vi "Documentation Application Tool.vi"() -> ()   [LabVIEW 2016]
uses:
  <vilib>/ni/Tree/Tree Manager/Tree.lvclass
  States.ctl
  <vilib>/ni/Tree/Data Types/String/String.lvclass/String.ctl
  <vilib>/ni/Tree/Data Types/String/To String Tree Data.vi
  <vilib>/ni/Tree/Data Types/String/From String Tree Data.vi
  <vilib>/ni/Tree/Data Types/String/String.lvclass
  C:/Program Files/National Instruments/LabVIEW 2016/vi.lib/ni/Tree/Tree Data/Tree Data.lvclass
  <vilib>/ni/Tree/Tree Manager/API/Set Attribute.vi
  <vilib>/ni/Tree/Tree Manager/API/Set Meta Data.vi
  <vilib>/ni/Tree/Tree Manager/API/Get Name.vi
  <vilib>/ni/Tree/Tree Manager/API/Set Name.vi
  <vilib>/ni/Tree/Tree Manager/API/Set Attribute Tree Data.vi
  <vilib>/xml/Load XML File.vi
  <vilib>/ni/Tree/Tree Manager/API/List Roots.vi
  <vilib>/ni/Tree/Tree Manager/API/Get Attribute Tree Data.vi
  <vilib>/ni/Tree/Tree Manager/API/Get Meta Data.vi
  <vilib>/ni/Tree/Tree Manager/API/Delete Attribute Tree Data.vi
  <vilib>/ni/Tree/Tree Manager/API/Get Attribute.vi
  <vilib>/xml/NI_XML.lvlib
panel:
  in  "Load XML File":bool
  in  "XML File Path":path=path "C:/Git/rfic-reference-design-libraries-csharp/CodeReport.xml"
  in  "Load Search Directory":bool
  in  "Search Directory":path=path "C:/Git/rf-adv-reference-design-libraries-labview/Source/SG"
  in  "Code Modules":string(tree)
  in  "XML File":string(tree)
  out "Selected Element":string
  in  "Element Description":string
  in  "Copy":bool
  out "Selected XML Data":string
  in  "Cancel":bool
  in  "Apply All Unsaved":bool
  in  "Cancel All":bool
  in  "Apply":bool
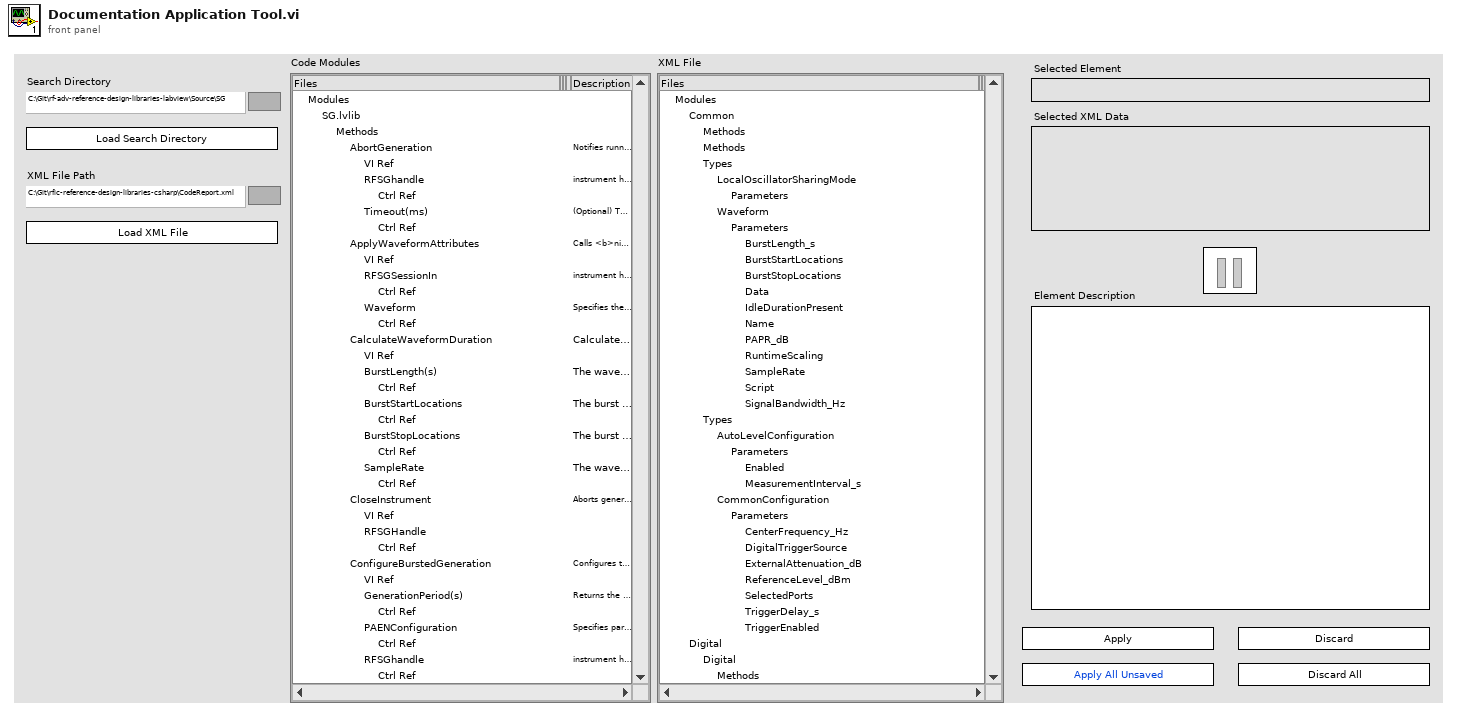
[diagram p1: front panel]
types:
  T1 = typedef "States.ctl" = enum16{"<Init>", "Wait for Event", "Update Code Modules Display", "Save Files", "<Shutdown>"}
  T2 = cluster{"LabVIEW Tree":refnum<data-value>, "XML Tree":refnum<data-value>, "References":refnum<vi>[], "Unsaved Items":variant, "Control Strings":string[], "Items to Save":string[]}
  T3 = enum32{"invalid VI type", "Standard VI", "Control VI", "Global VI", "Polymorphic VI", "Configuration VI", "SubSystem", "Facade VI", "Method VI", "Statechart Diagram VI"}
  T4 = enum16{"Left Button", "Center Button", "Right Button", "Window Close"}
  T5 = cluster{"Left Cell String":string, "Child Text":string[], "Child Tag":string, "Item Indent":i32, "Child Only?":bool, "Glyph Index":i32}[]
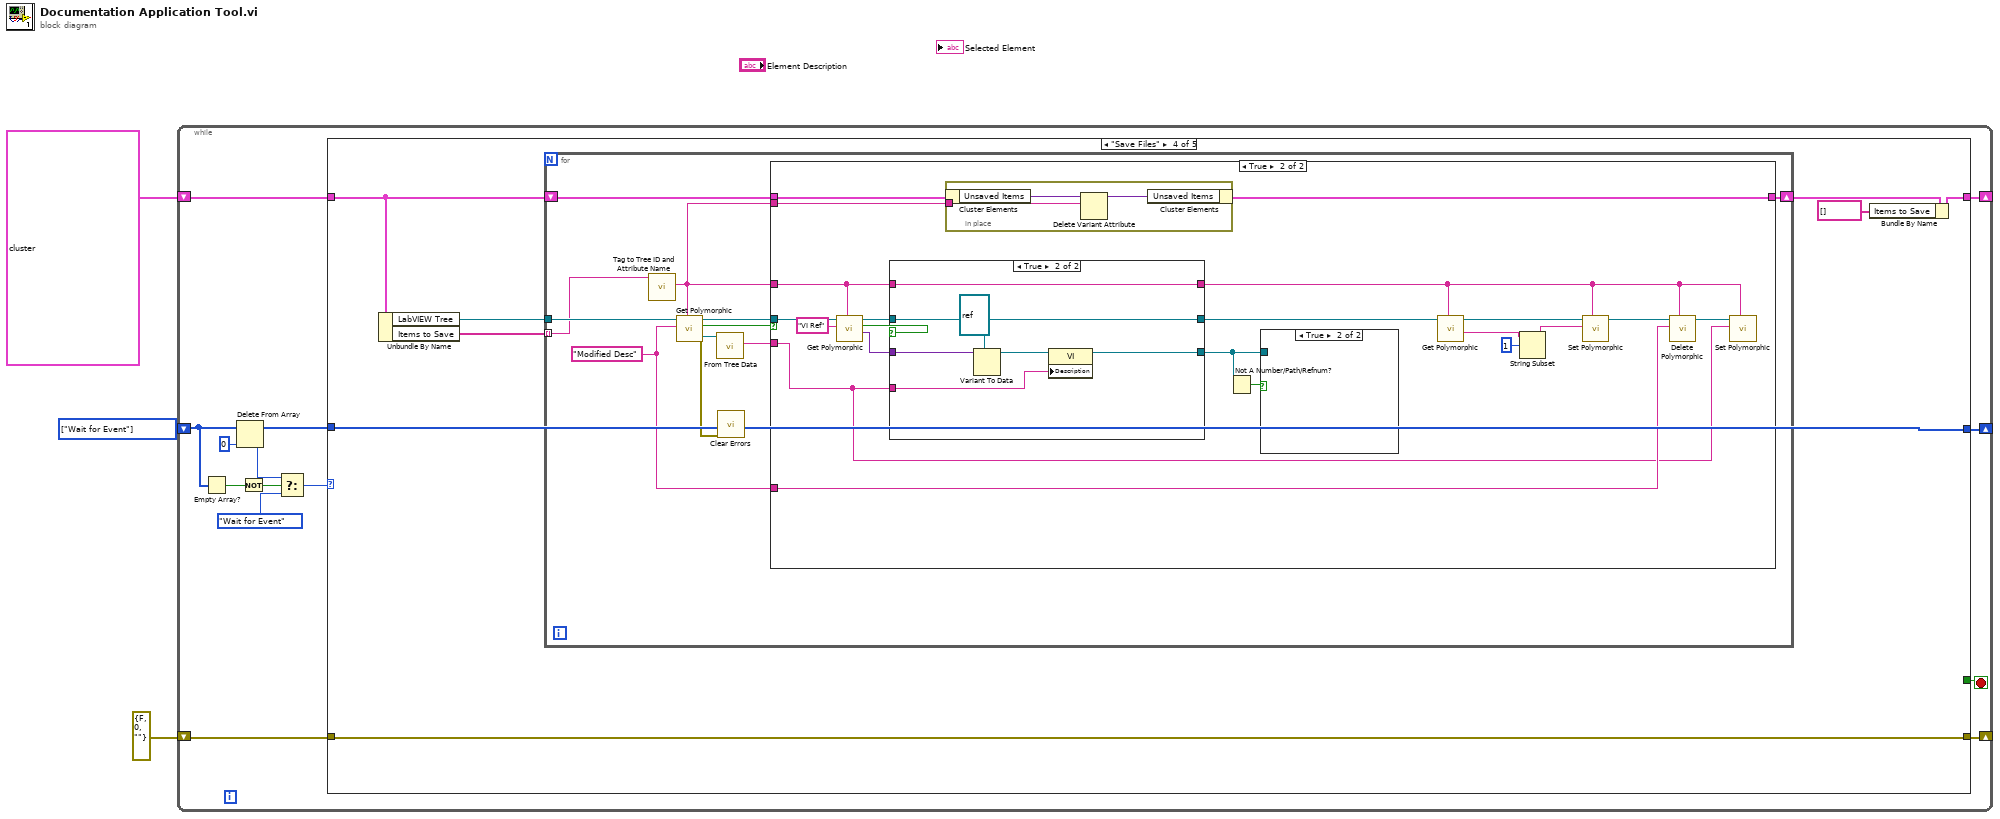
[diagram p0: block diagram]
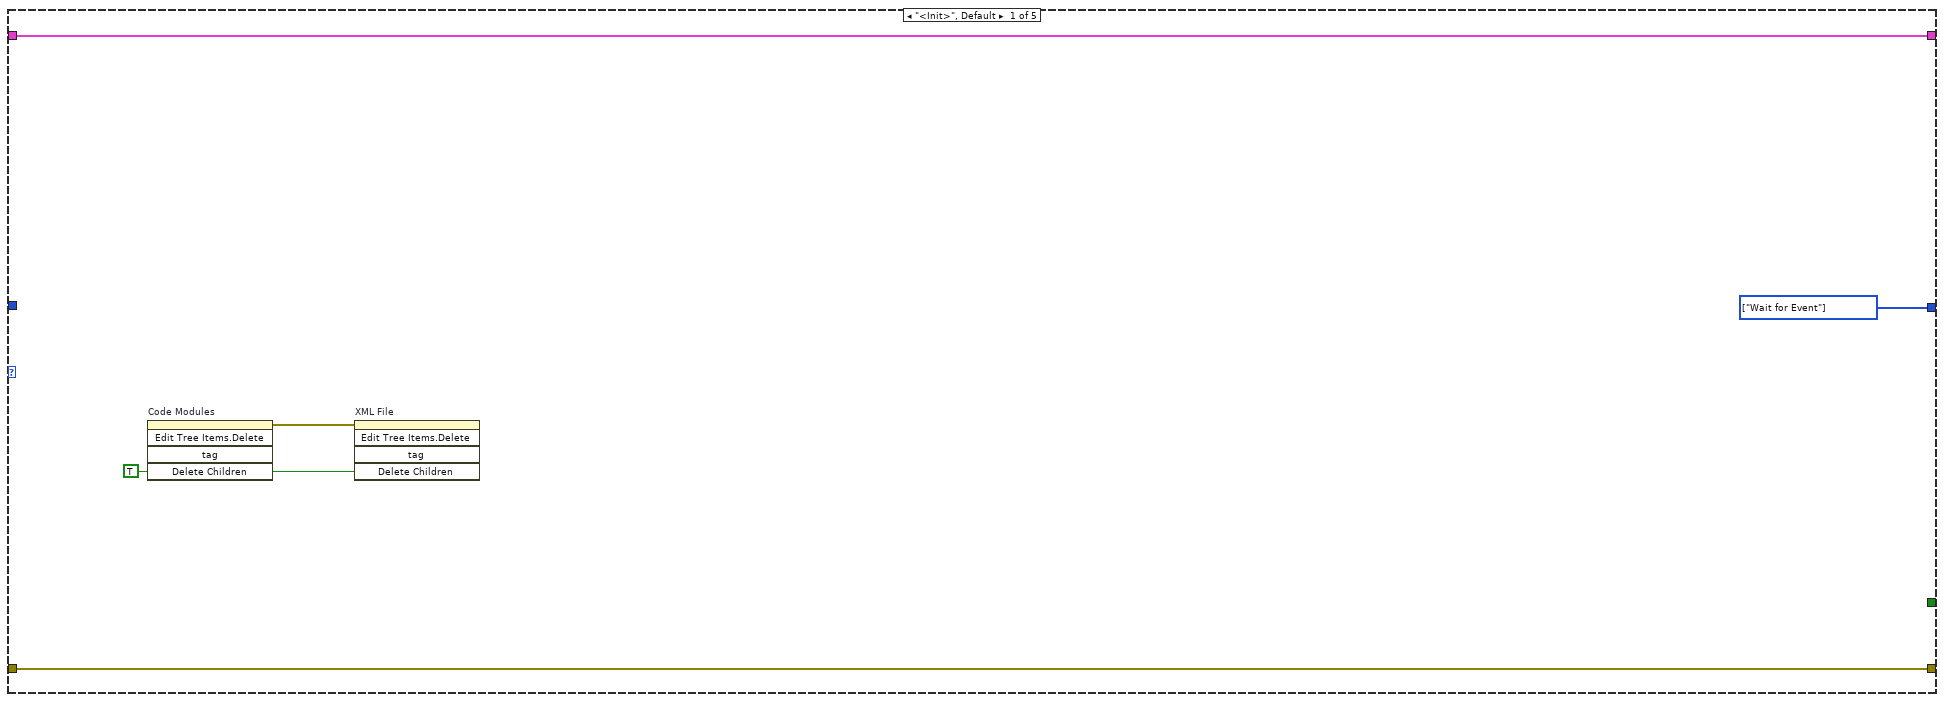
[diagram p2: hidden frame]
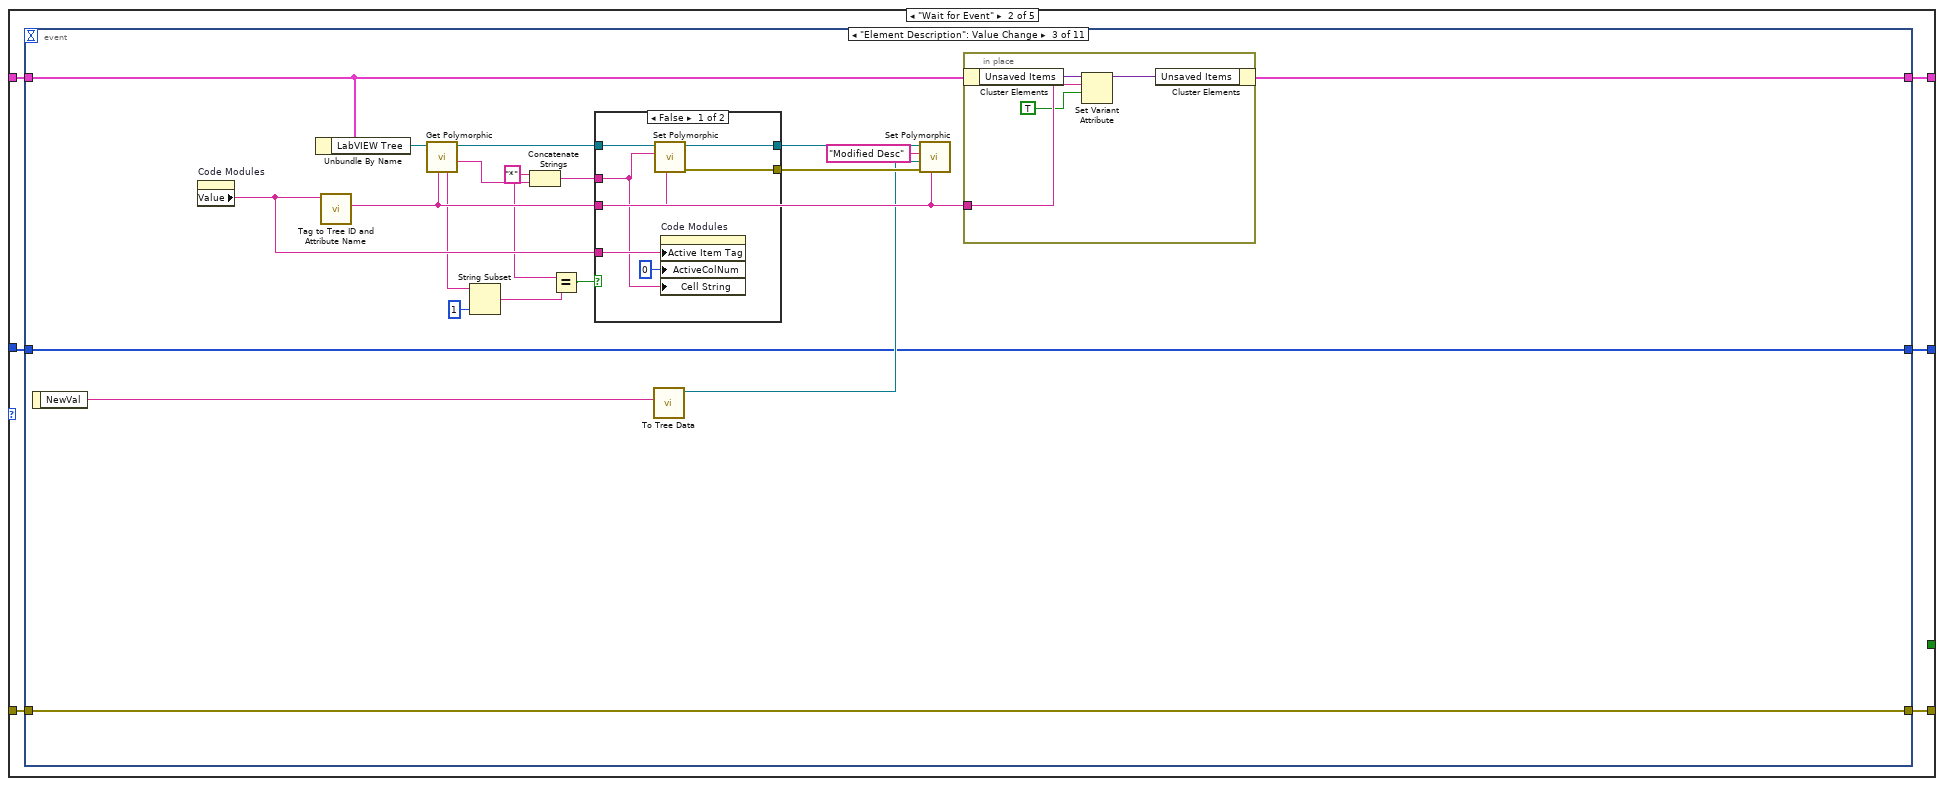
[diagram p3: hidden frame]
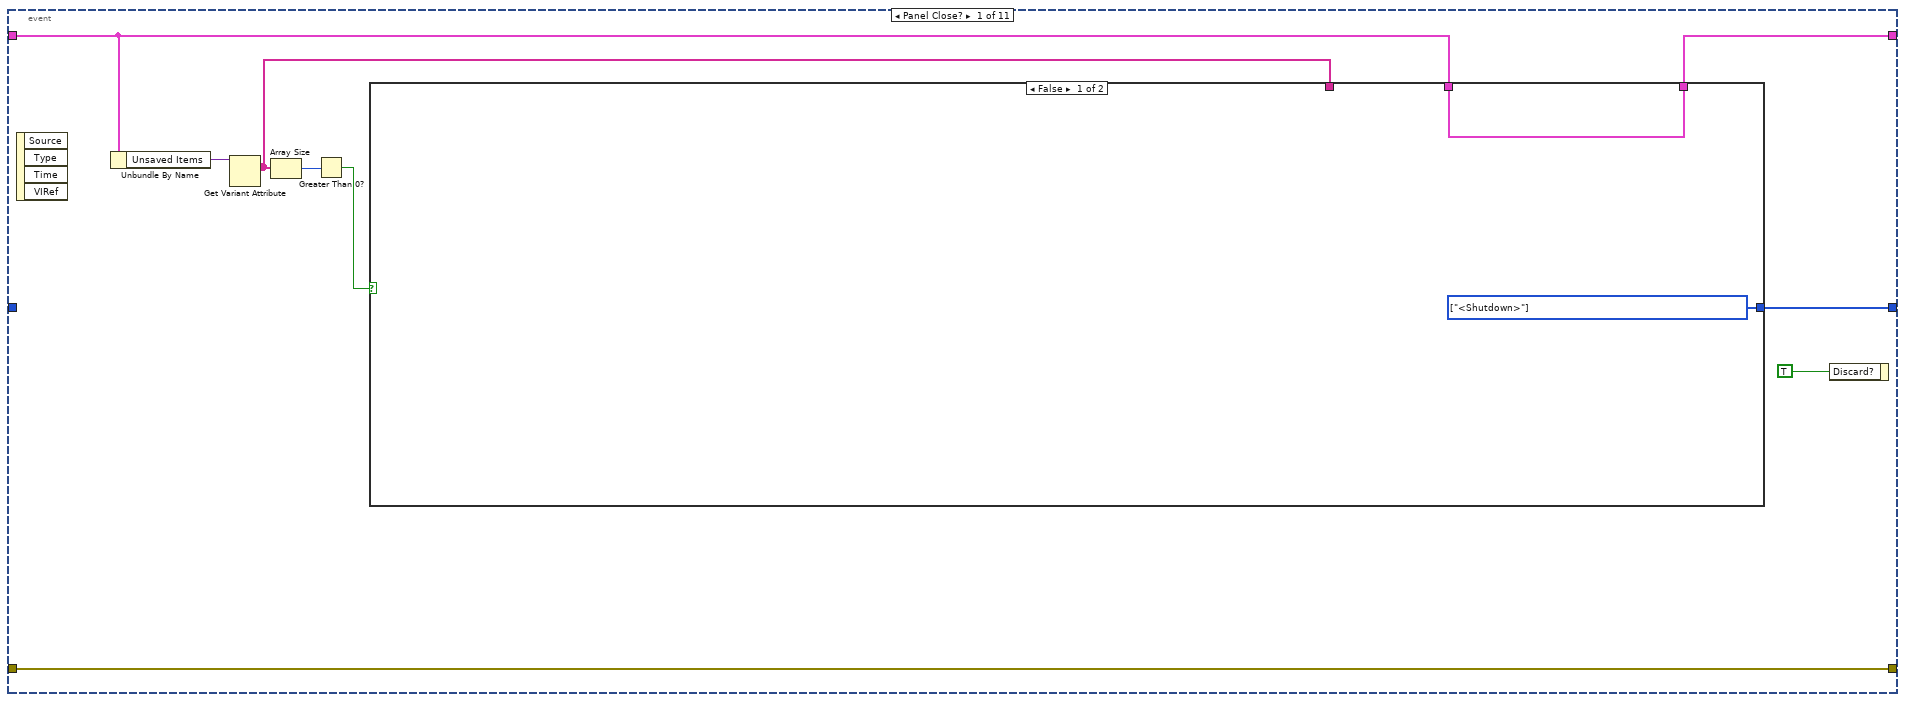
[diagram p4: hidden frame]
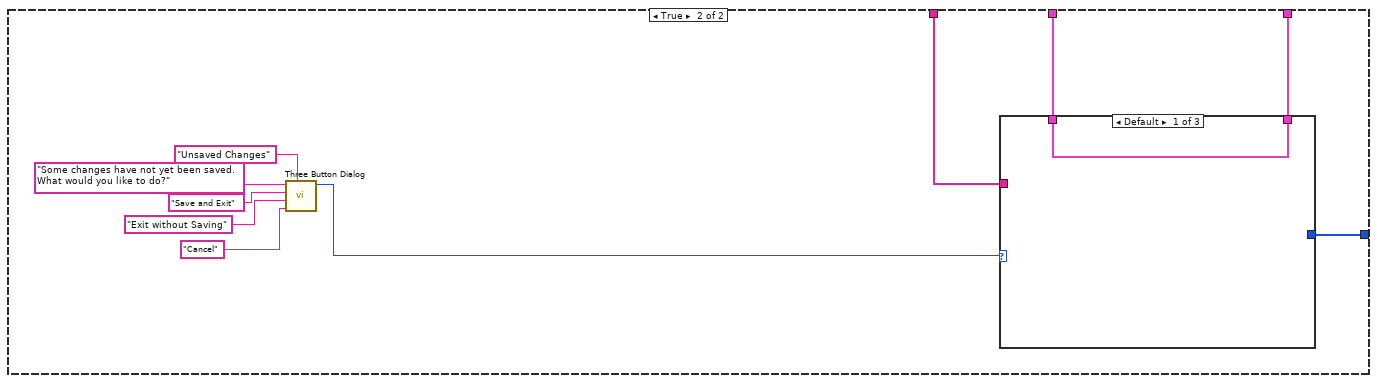
[diagram p5: hidden frame]
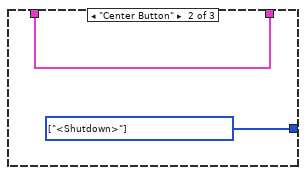
[diagram p6: hidden frame]
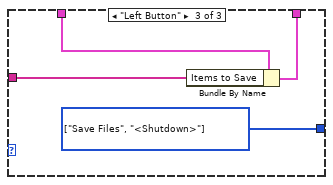
[diagram p7: hidden frame]
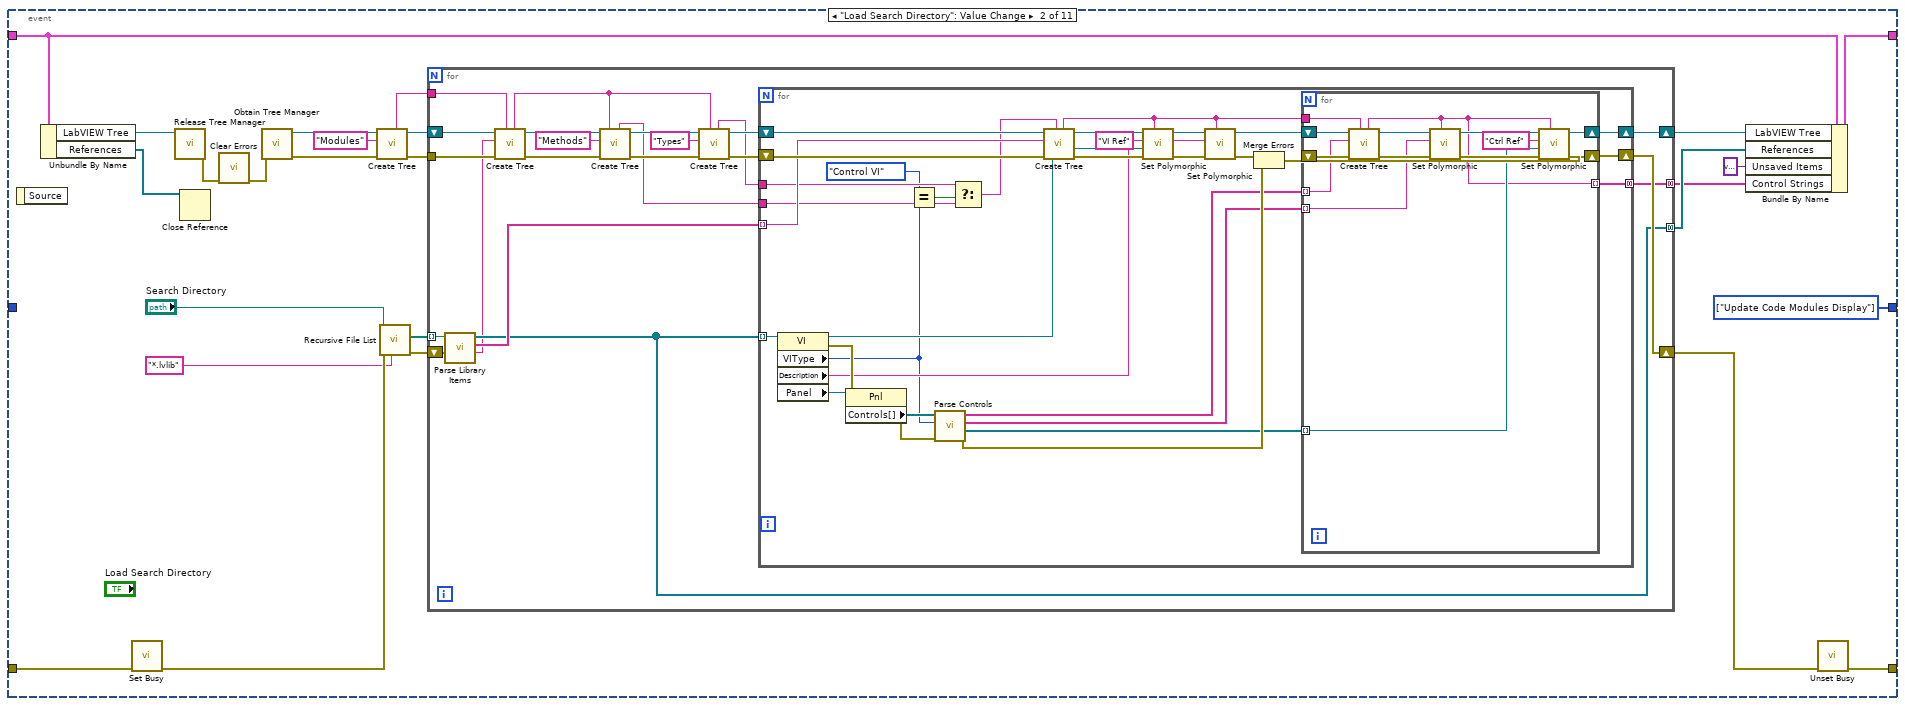
[diagram p8: hidden frame]
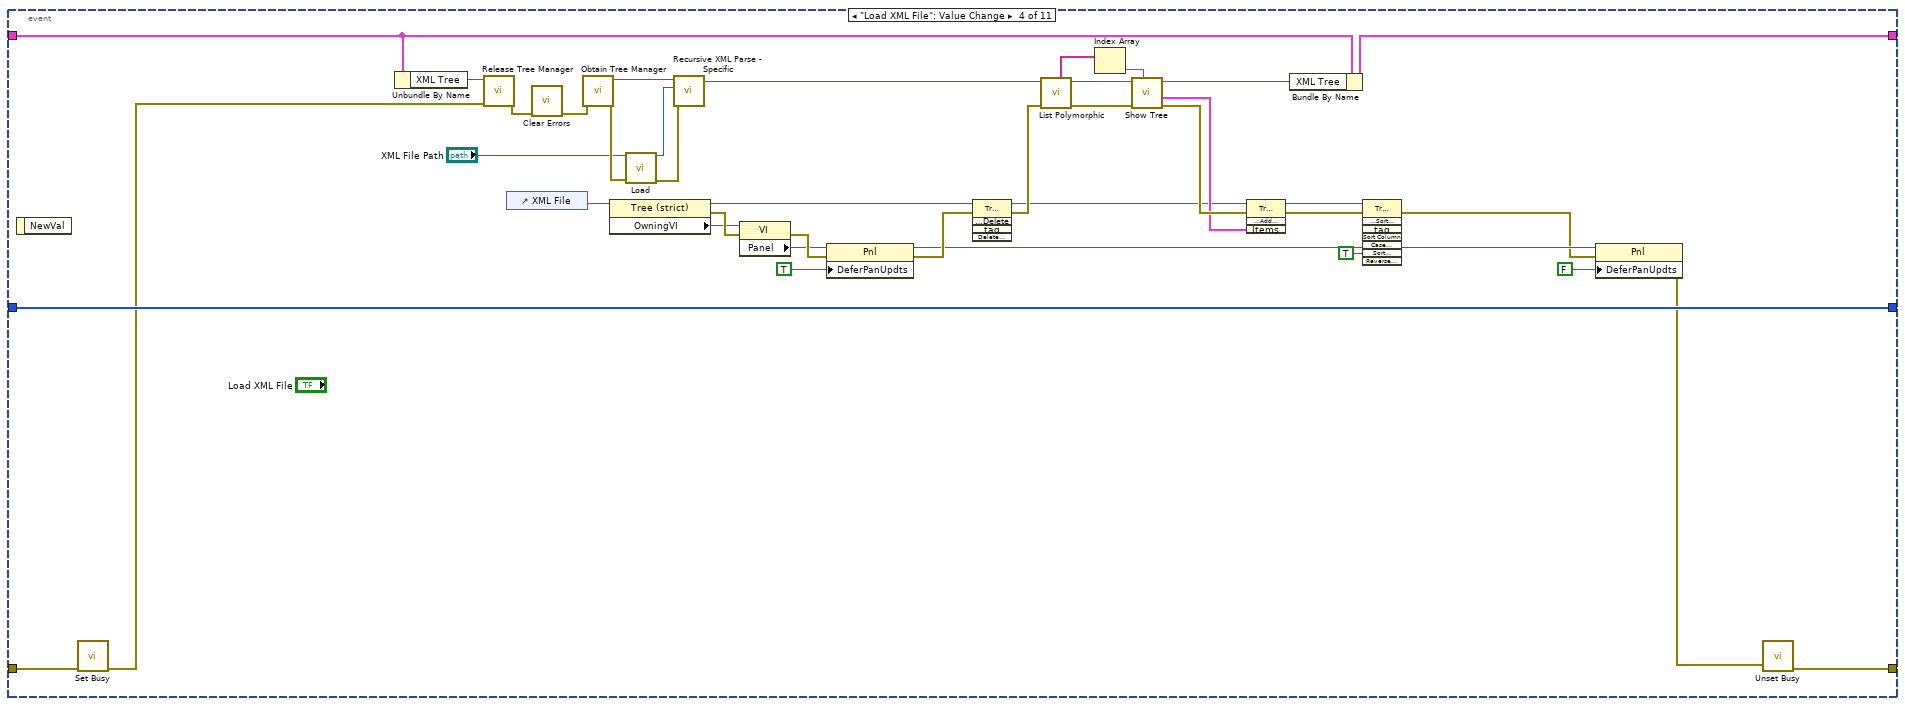
[diagram p10: hidden frame]
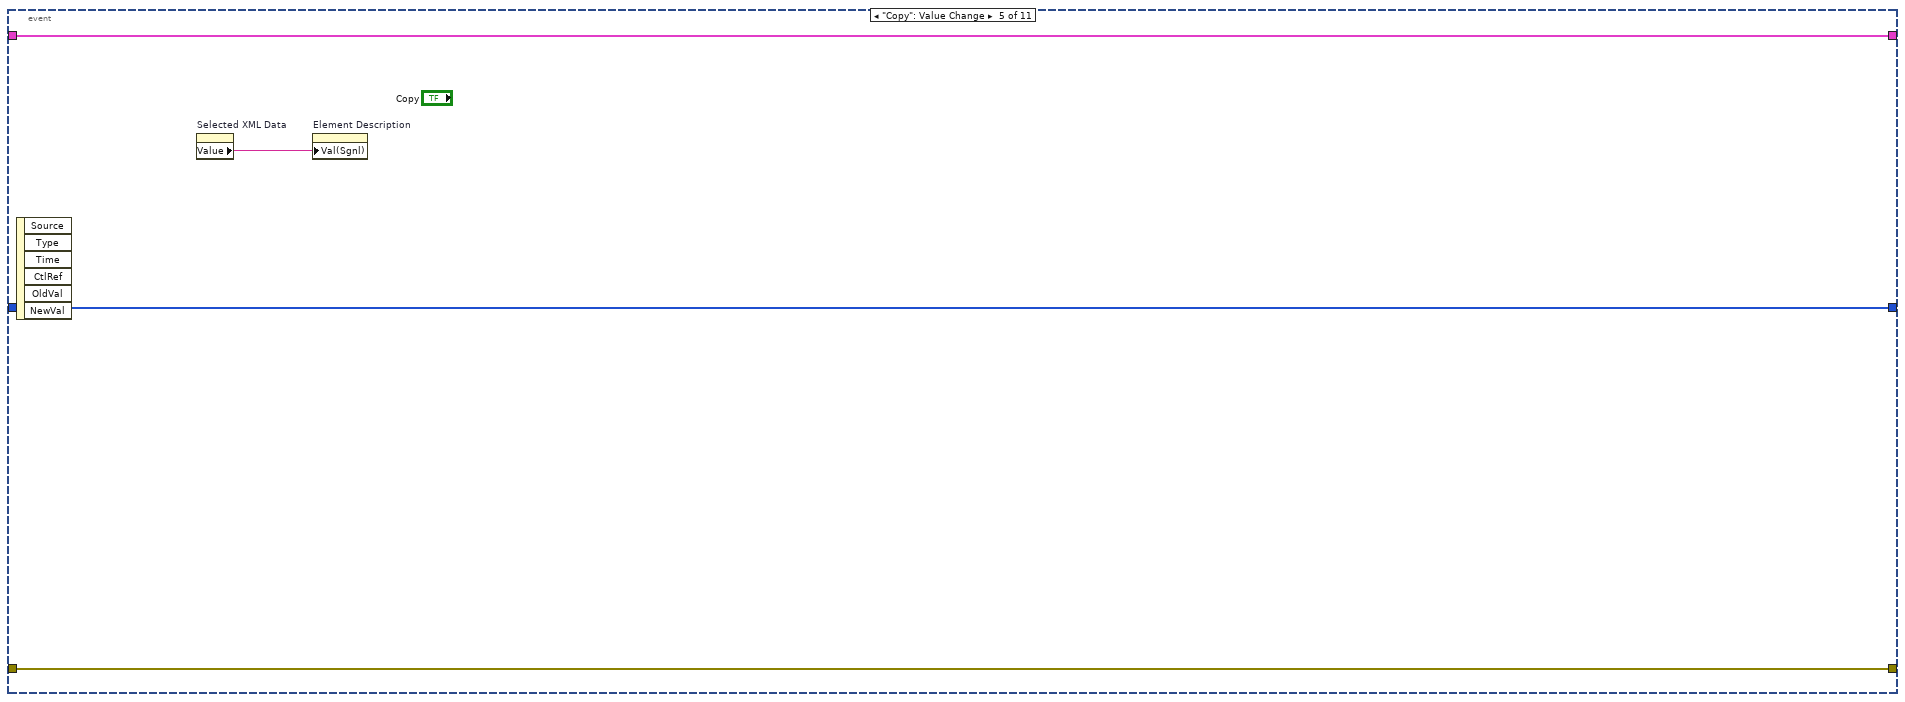
[diagram p11: hidden frame]
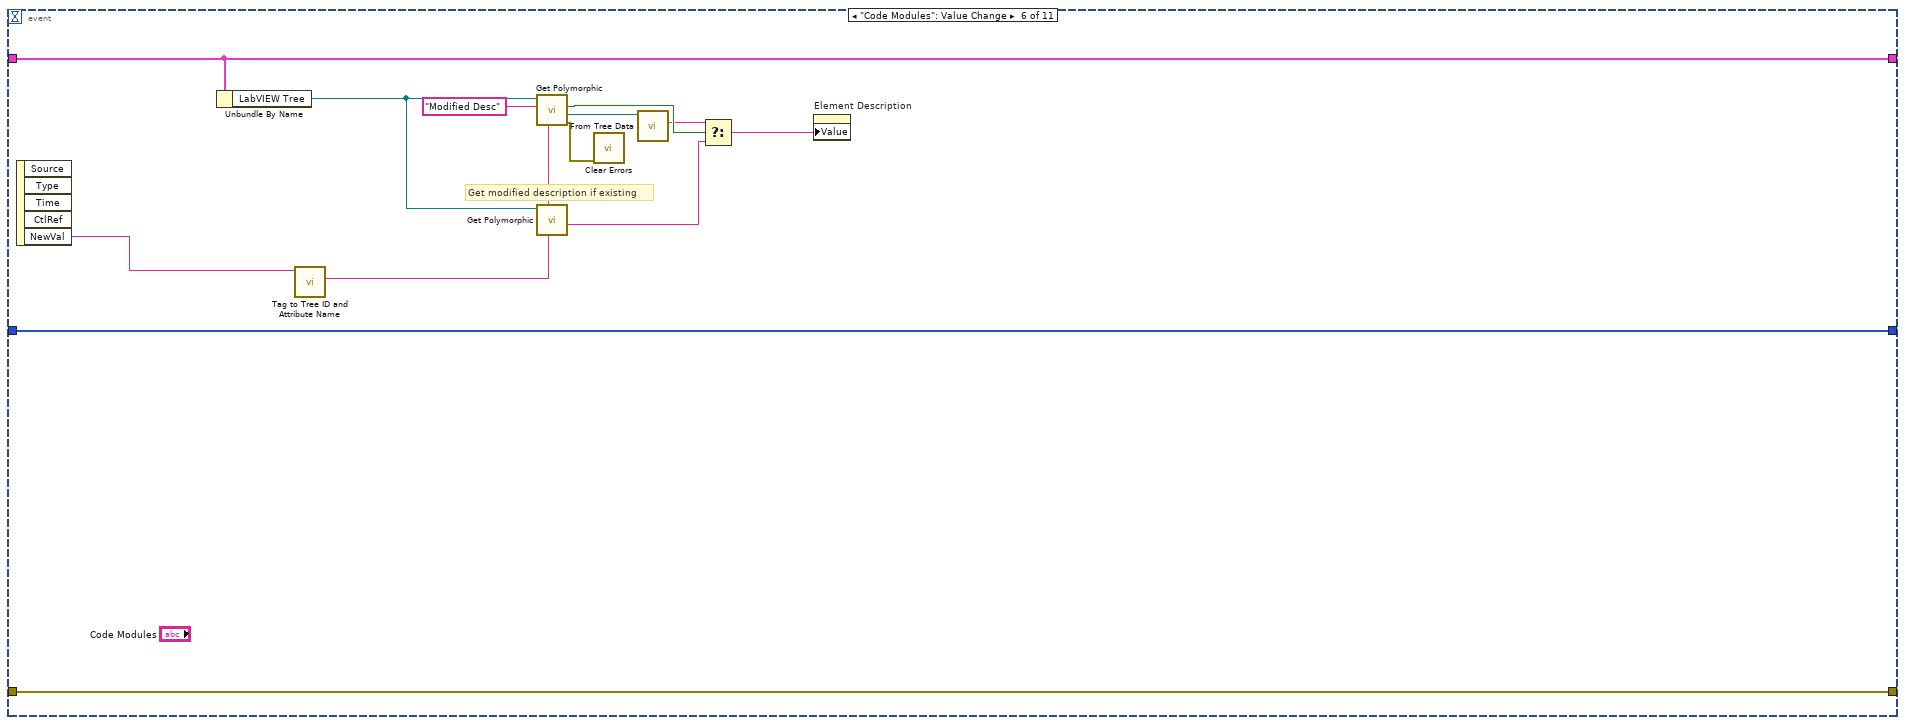
[diagram p12: hidden frame]
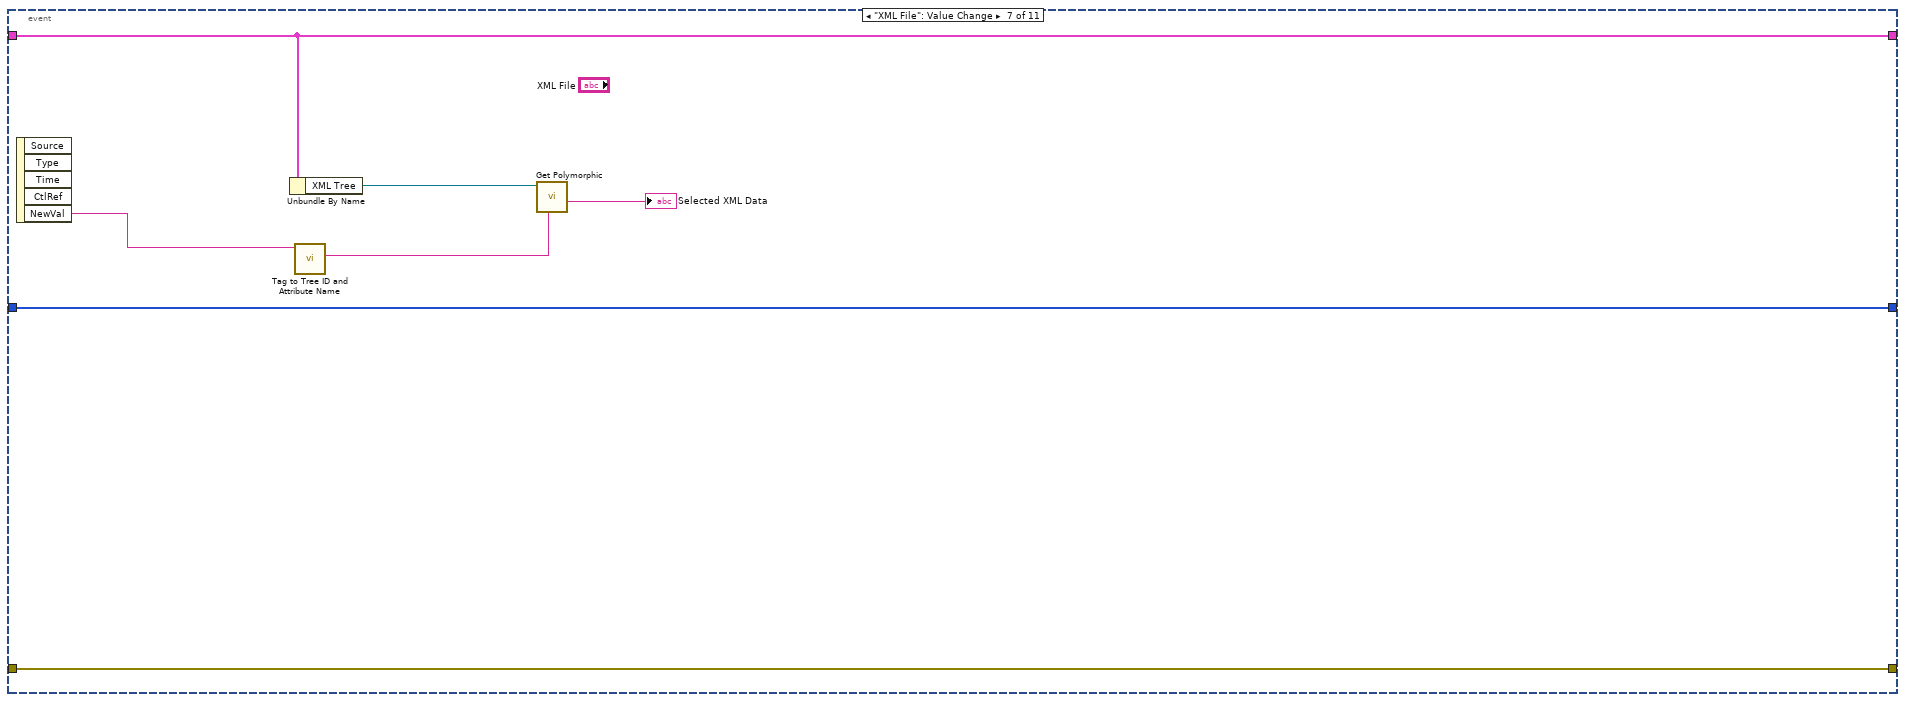
[diagram p13: hidden frame]
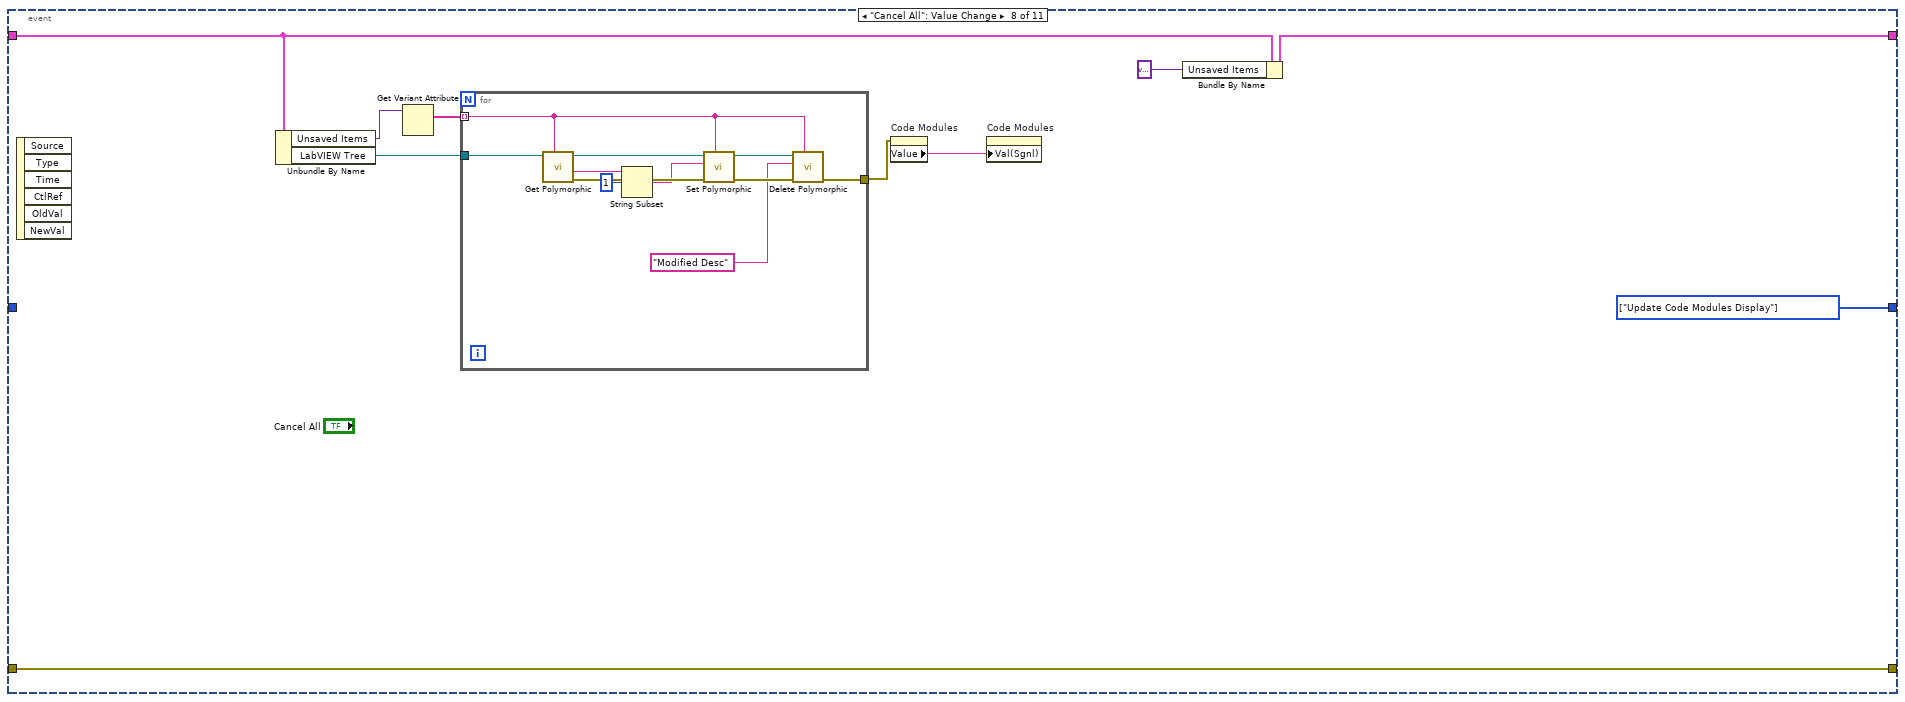
[diagram p14: hidden frame]
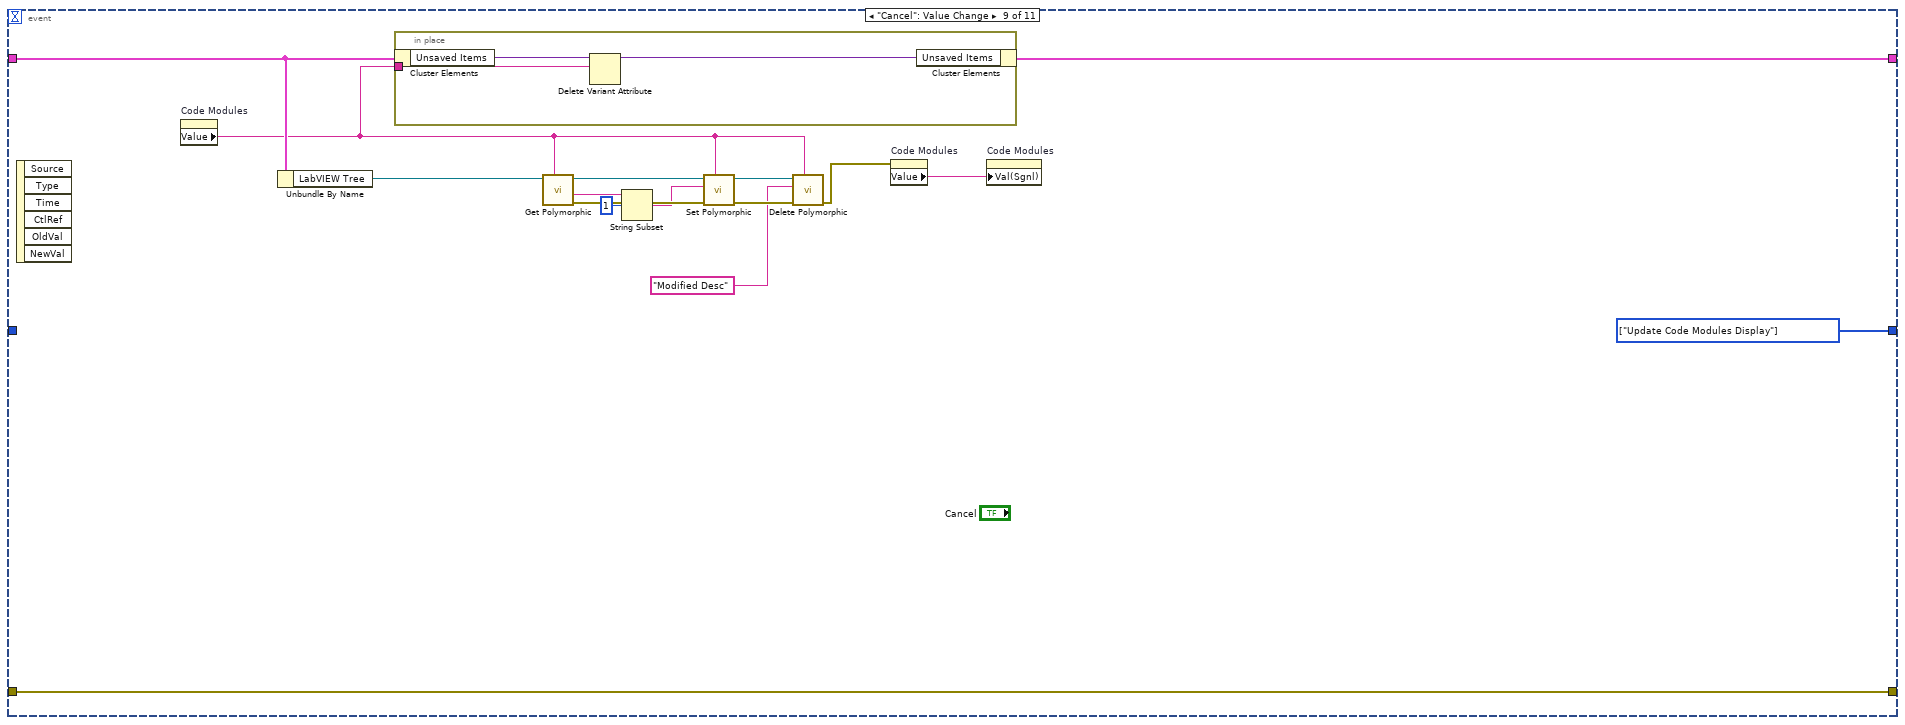
[diagram p15: hidden frame]
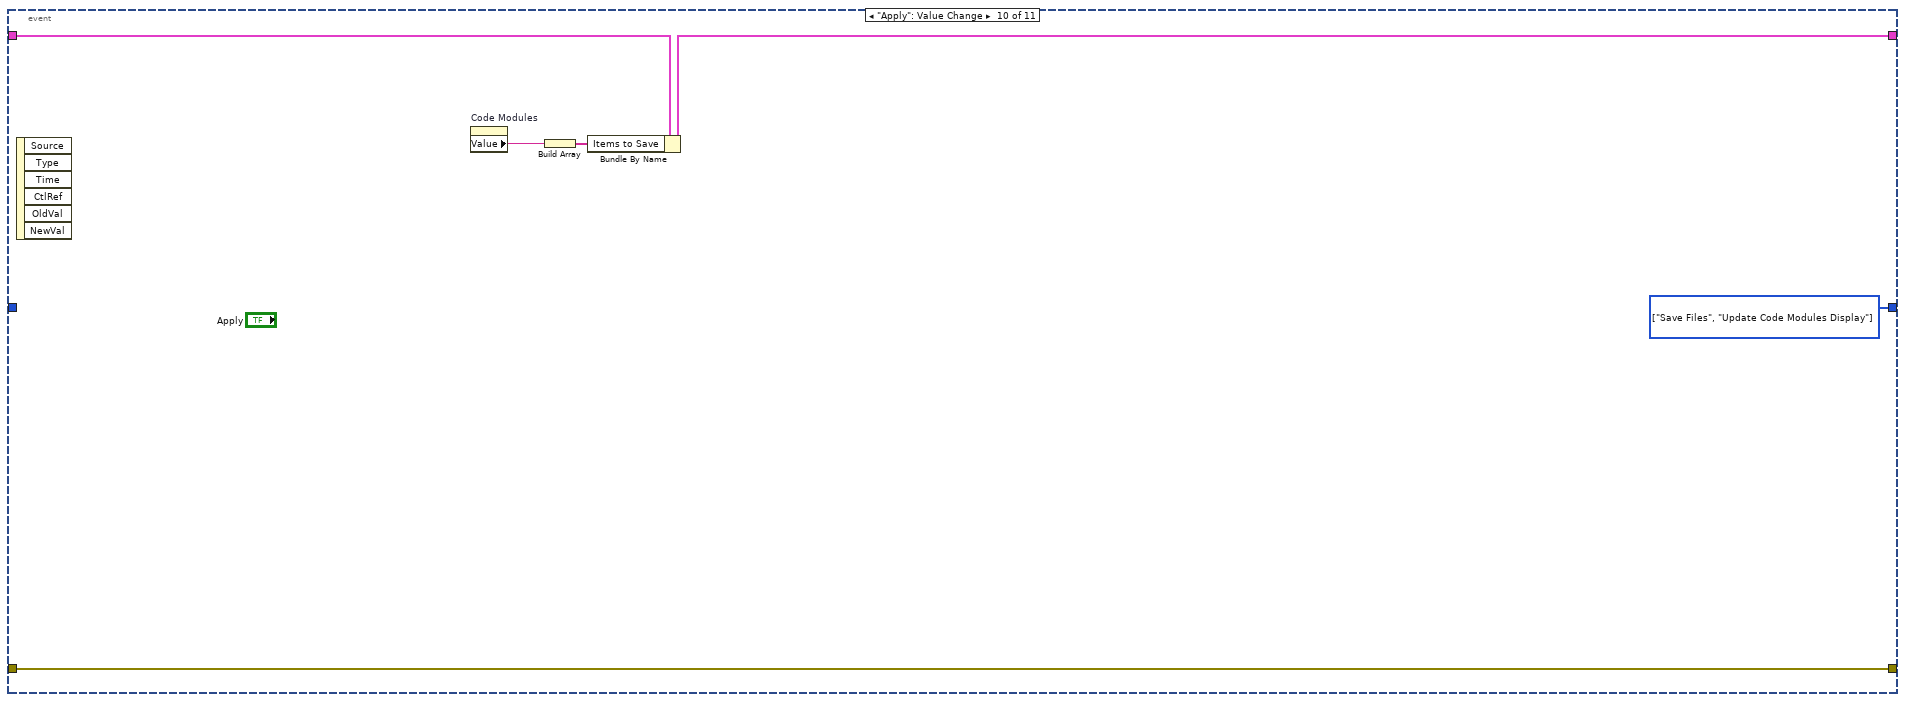
[diagram p16: hidden frame]
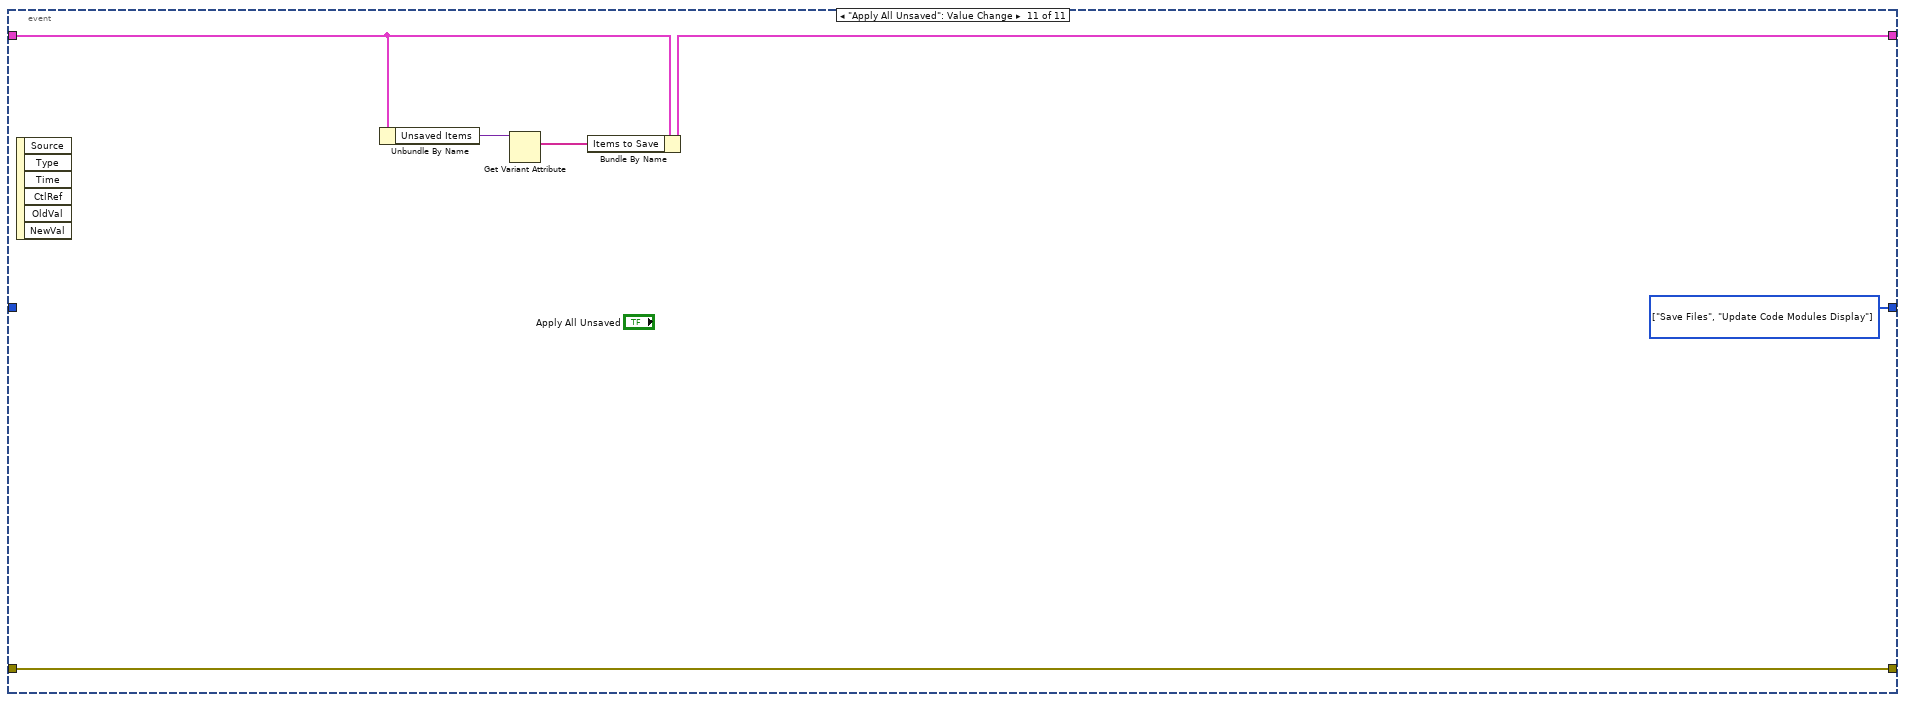
[diagram p17: hidden frame]
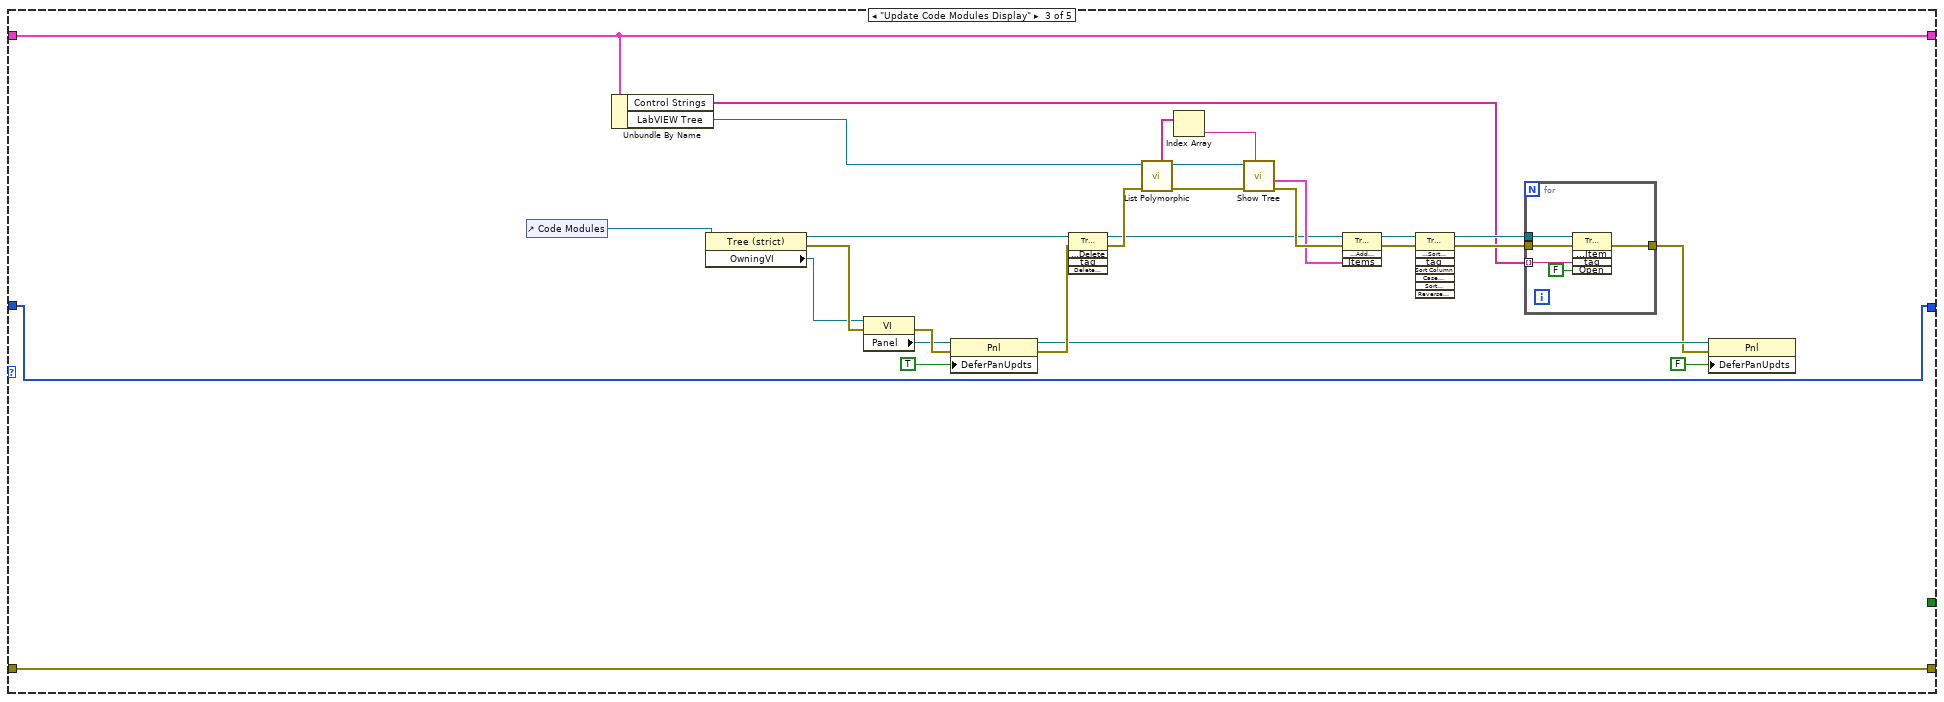
[diagram p18: hidden frame]
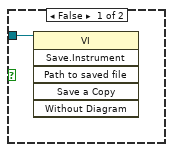
[diagram p20: hidden frame]
diagram:
  w1 = T1[] [enum."Wait for Event"] items=["<Init>", "Wait for Event", "Update Code Modules Display", "Save Files", "<Shutdown>"]
  n1 = while {
    shift-right: [w16] -> _
    shift-left: errorcluster {"status"=FALSE, "code"=0, "source"=""} ("error constant") -> [w17]
    shift-right: [w14] -> _
    shift-left: T2 {"LabVIEW Tree"=refnum, "XML Tree"=refnum, "References"=[], "Unsaved Items"=variant, "Control Strings"=[], "Items to Save"=[]} -> [w15]
    shift-right: [w5] -> _
    shift-left: w1 -> [w11]
    stop <- w4 stop-if-true
    n2 = Empty Array?(array=w11) -> (empty?=w10:bool)
    n3 = Delete From Array(array=w11, index=0) -> (deleted portion=w9:T1, array with subset deleted=w13:T1[])  [unwired: 1 in]
    n4 = Not(x=w10) -> (.not. x?=w8:bool)
    n5 = Select(t=w9, s=w8, f=States."Wait for Event") -> (s? t:f=w6:T1)
    n6 = case shown="\"Save Files\"" w6 {
      tunnel: w17 -> [w21 w28 w323 w336 w404]
      tunnel: [w21 w27 w323 w336 w404] -> w16
      tunnel: w15 -> [w18 w26 w315 w334 w401]
      tunnel: [w18 w25 w315 w331 w401] -> w14
      tunnel: w13 -> [_ w23 w296 w329 w402]
      tunnel: [w19 w24 w296 w329 w402] -> w5
      tunnel: [_ _ _ _ TRUE] -> w4
      frame "<Init>", Default {
        w19 = T1[] [enum."Wait for Event"] items=["<Init>", "Wait for Event", "Update Code Modules Display", "Save Files", "<Shutdown>"]
        w20 = TRUE ("Delete Children?")
        n7 = invoke on="Code Modules" class="Tree (strict)" method="Edit Tree Items.Delete"("Delete Children"=w20) -> (error out=w22:errorcluster)  [unwired: 4 in, 4 out]
        n8 = invoke on="XML File" class="Tree (strict)" method="Edit Tree Items.Delete"(error in=w22, "Delete Children"=w20) -> ()  [unwired: 3 in, 5 out]
      }
      frame "Wait for Event" {
        n9 = event shown="[2] \"Element Description\": Value Change" {
          selector: _ -> [_ _ _ _ _ _ _ _ _ _ _]
          dyn-events: _ -> [_ _ _ _ _ _ _ _ _ _ _]
          timeout: _ -> [_ _ _ _ _ _ _ _ _ _ _]
          tunnel: w28 -> [w37 w80 w168 w219 w223 w236 w243 w253 w280 w289 w295]
          tunnel: [w37 w79 w168 w186 w223 w236 w243 w253 w280 w289 w295] -> w27
          tunnel: w26 -> [w32 w63 w163 w205 w222 w235 w242 w252 w267 w287 w292]
          tunnel: [w31 w64 w162 w206 w222 w235 w242 w245 w265 w286 w293] -> w25
          tunnel: [w35 w60 w150 w188 w220 w224 w237 w250 w278 w288 w294] -> w24
          tunnel: w23 -> [_ _ w150 w188 w220 w224 w237 _ _ _ _]
          event Panel Close? {
            n10 = event-data() -> ()  [unwired: 1 in, 4 out]
            n11 = Unbundle By Name(w32) -> ("Unsaved Items"=w34:variant)
            n12 = Get Variant Attribute(Variant=w34) -> (names=w30:string[])  [unwired: 3 in, 3 out]
            n13 = Array Size(array=w30) -> (size(s)=w33:i32)
            n14 = Greater Than 0?(x=w33) -> (x > 0?=w29:bool)
            n15 = case shown="False" w29 {
              tunnel: [w38 w49] -> w35
              tunnel: w32 -> [w39 w47]
              tunnel: [w39 w46] -> w31
              tunnel: w30 -> [_ w45]
              frame False {
                w38 = T1[] [enum."<Shutdown>"] items=["<Init>", "Wait for Event", "Update Code Modules Display", "Save Files", "<Shutdown>"]
              }
              frame True {
                n16 = call <vilib>:"Three Button Dialog.vi"("Window Title (\"\")"="Unsaved Changes" ("Window Title (\"\")"), "Right Button Text (\"Cancel\")"="Cancel" ("Right Button Text (\"Cancel\")"), "Center Button Text (\"No\")"="Exit without Saving" ("Center Button Text (\"No\")"), "Left Button Text (\"Yes\")"="Save and Exit" ("Left Button Text (\"Yes\")"), "message"="Some changes have not yet been saved. What would you like to do?") -> ("Which Button?"=w48:T4)  [unwired: 6 in]
                n17 = case shown="Default" w48 {
                  tunnel: [_ w52 w56] -> w49
                  tunnel: w47 -> [w50 w51 w55]
                  tunnel: [w50 w51 w54] -> w46
                  tunnel: w45 -> [_ _ w53]
                  frame Default {
                  }
                  frame "Center Button" {
                    w52 = T1[] [enum."<Shutdown>"] items=["<Init>", "Wait for Event", "Update Code Modules Display", "Save Files", "<Shutdown>"]
                  }
                  frame "Left Button" {
                    w56 = T1[] [enum."Save Files", enum."<Shutdown>"] items=["<Init>", "Wait for Event", "Update Code Modules Display", "Save Files", "<Shutdown>"]
                    n18 = Bundle By Name(cluster=w55, "Items to Save"=w53) -> (w54:T2)
                  }
                }
              }
            }
            n19 = event-data("Discard?"=TRUE) -> ()  [unwired: 1 in, 1 out]
          }
          event "Load Search Directory": Value Change {
            w60 = T1[] [enum."Update Code Modules Display"] items=["<Init>", "Wait for Event", "Update Code Modules Display", "Save Files", "<Shutdown>"]
            n20 = event-data() -> ()  [unwired: 1 in, 1 out]
            n21 = Unbundle By Name(w63) -> ("LabVIEW Tree"=w69:refnum<data-value>, "References"=w59:refnum<vi>[])
            n22 = call <vilib>:"Set Busy.vi"("error in (no error)"=w80) -> ("error out"=w74:errorcluster)  [unwired: 9 in, 1 out]
            n23 = call <vilib>:"Release Tree Manager.vi"("Tree"=w69) -> ("Error Out"=w78:errorcluster)  [unwired: 10 in]
            n24 = Close Reference(reference=w59) -> ()  [unwired: 1 in, 1 out]
            n25 = call <vilib>:"Clear Errors.vi"("error in (no error)"=w78) -> ("error out"=w77:errorcluster)  [unwired: 5 in, 1 out]
            n26 = call <vilib>:"Obtain Tree Manager.vi"("Error In"=w77) -> ("Error Out"=w76:errorcluster, "Tree"=w68:refnum<data-value>)  [unwired: 9 in]
            n27 = call <vilib>:"Create Tree.vi"("Error In"=w76, "Name"="Modules", "Tree Manager"=w68) -> ("Error Out"=w75:errorcluster, "Tree Manager"=w65:refnum<data-value>, "Unique ID"=w66:string)  [unwired: 6 in]
            n28 = call <vilib>:"Recursive File List.vi"("pattern"="*.lvlib", "error in (no error)"=w74, "Folder Path"="Search Directory") -> ("error out"=w81:errorcluster, "All Files in Dir"=w70:path[])  [unwired: 4 in, 3 out]
            n29 = for {
              tunnel: w70 -> [w97] mode=indexing
              shift-right: [w98] -> w73
              shift-left: w81 -> [w103]
              tunnel: w66 -> [w92]
              tunnel: w75 -> [w102]
              tunnel: [w95] -> w62 mode=concatenating
              shift-right: [w83] -> w61
              shift-left: w65 -> [w94]
              tunnel: [w82] -> w57 mode=concatenating
              n30 = call "Parse Library Items.vi"("error in (no error)"=w103, "Library Path"=w97) -> ("Display Name"=w93:string, "File Names"=w96:string[], "References"=w95:refnum<vi>[])  [unwired: 6 in, 1 out]
              n31 = call <vilib>:"Create Tree.vi"("Parent ID (empty)"=w92, "Error In"=w102, "Name"=w93, "Tree Manager"=w94) -> ("Error Out"=w101:errorcluster, "Tree Manager"=w90:refnum<data-value>, "Unique ID"=w91:string)  [unwired: 5 in]
              n32 = call <vilib>:"Create Tree.vi"("Parent ID (empty)"=w91, "Error In"=w101, "Name"="Methods", "Tree Manager"=w90) -> ("Error Out"=w100:errorcluster, "Tree Manager"=w89:refnum<data-value>, "Unique ID"=w85:string)  [unwired: 5 in]
              n33 = call <vilib>:"Create Tree.vi"("Parent ID (empty)"=w91, "Error In"=w100, "Name"="Types", "Tree Manager"=w89) -> ("Error Out"=w99:errorcluster, "Tree Manager"=w86:refnum<data-value>, "Unique ID"=w84:string)  [unwired: 5 in]
              n34 = for {
                tunnel: w95 -> [w126] mode=indexing
                tunnel: w96 -> [w120] mode=indexing
                tunnel: w85 -> [w117]
                tunnel: w84 -> [w118]
                shift-right: [w107] -> w83
                shift-left: w86 -> [w121]
                shift-right: [w127] -> w98
                shift-left: w99 -> [w134]
                tunnel: [w104] -> w82 mode=concatenating
                n35 = property class="VI"(reference=w126) -> (reference out=w112:refnum<vi>, error out=w135:errorcluster, "VIType"=w105:T3, "Description"=w114:string, "Panel"=w106:refnum<vi>)  [unwired: 1 in]
                n36 = property class="Pnl"(reference=w106, error in=w135) -> (error out=w130:errorcluster, "Controls[]"=w125:refnum<vi>[])  [unwired: 1 out]
                n37 = Equal?(x=T3."Control VI" ("y"), y=w105) -> (x = y?=w119:bool)
                n38 = call "Parse Controls.vi"("error in (no error)"=w130, "VI Type"=w105, "Controls[]"=w125) -> ("error out"=w128:errorcluster, "References"=w122:refnum<vi>[], "Control Descriptions"=w123:string[], "Control Names"=w124:string[])  [unwired: 5 in]
                n39 = Select(t=w118, s=w119, f=w117) -> (s? t:f=w115:string)
                n40 = call <vilib>:"Create Tree.vi"("Parent ID (empty)"=w115, "Error In"=w134, "Name"=w120, "Tree Manager"=w121) -> ("Error Out"=w133:errorcluster, "Tree Manager"=w111:refnum<data-value>, "Unique ID"=w108:string)  [unwired: 5 in]
                n41 = call-poly <vilib>:"Set Polymorphic.vi"("Tree ID"=w108, "Error In"=w133, "Attribute Value"=w112, "Attribute Name"="VI Ref", "Tree Manager"=w111) -> ("Error Out"=w132:errorcluster, "Tree Manager"=w110:refnum<data-value>)  [unwired: 4 in, 1 out]
                n42 = call-poly <vilib>:"Set Polymorphic.vi"("Tree ID"=w108, "Error In"=w132, "Meta Data"=w114, "Tree Manager"=w110) -> ("Error Out"=w131:errorcluster, "Tree Manager"=w109:refnum<data-value>)  [unwired: 6 in]
                n43 = Merge Errors(w131, w128) -> (w129:errorcluster)
                n44 = for {
                  tunnel: w124 -> [w143] mode=indexing
                  tunnel: w123 -> [w142] mode=indexing
                  tunnel: w122 -> [w137] mode=indexing
                  shift-right: [w146] -> w127
                  shift-left: w129 -> [w149]
                  tunnel: w108 -> [w144]
                  shift-right: [w139] -> w107
                  shift-left: w109 -> [w145]
                  tunnel: [w136] -> w104 mode=indexing
                  n45 = call <vilib>:"Create Tree.vi"("Parent ID (empty)"=w144, "Error In"=w149, "Name"=w143, "Tree Manager"=w145) -> ("Error Out"=w148:errorcluster, "Tree Manager"=w141:refnum<data-value>, "Unique ID"=w136:string)  [unwired: 5 in]
                  n46 = call-poly <vilib>:"Set Polymorphic.vi"("Tree ID"=w136, "Error In"=w148, "Meta Data"=w142, "Tree Manager"=w141) -> ("Error Out"=w147:errorcluster, "Tree Manager"=w140:refnum<data-value>)  [unwired: 6 in]
                  n47 = call-poly <vilib>:"Set Polymorphic.vi"("Tree ID"=w136, "Error In"=w147, "Attribute Value"=w137, "Attribute Name"="Ctrl Ref", "Tree Manager"=w140) -> ("Error Out"=w146:errorcluster, "Tree Manager"=w139:refnum<data-value>)  [unwired: 4 in, 1 out]
                }
              }
            }
            n48 = Bundle By Name(cluster=w63, "LabVIEW Tree"=w61, "References"=w62, "Unsaved Items"=variant, "Control Strings"=w57) -> (w64:T2)
            n49 = call <vilib>:"Unset Busy.vi"("error in (no error)"=w73) -> ("error out"=w79:errorcluster)  [unwired: 10 in]
          }
          event "Element Description": Value Change {
            w152 = "*" ("string")
            n50 = event-data() -> ("NewVal"=w158:string)  [unwired: 1 in]
            n51 = property on="Code Modules" class="Tree (strict)"() -> ("Value"=w164:string)  [unwired: 2 in, 2 out]
            n52 = Unbundle By Name(w163) -> ("LabVIEW Tree"=w166:refnum<data-value>)
            n53 = call <vilib>:"Tag to Tree ID and Attribute Name.vi"("Tag"=w164) -> ("Tree ID"=w160:string)  [unwired: 8 in, 2 out]
            n54 = call-poly <vilib>:"Get Polymorphic.vi"("Tree ID"=w160, "Tree Manager"=w166) -> ("Name"=w156:string, "Tree Manager"=w165:refnum<data-value>)  [unwired: 7 in, 1 out]
            n55 = String Subset(string=w156, length (rest)=1 ("length (rest)")) -> (substring=w153:string)  [unwired: 1 in]
            n56 = Concatenate Strings(w152, w156) -> (w154:string)
            n57 = Equal?(x=w152, y=w153) -> (x = y?=w151:bool)
            n58 = case shown="False" w151 {
              tunnel: [w175 _] -> w167
              tunnel: w165 -> [w174 w176]
              tunnel: w164 -> [w173 _]
              tunnel: [w171 w176] -> w161
              tunnel: w160 -> [w170 _]
              tunnel: w154 -> [w169 _]
              frame False {
                n59 = call-poly <vilib>:"Set Polymorphic.vi"("Tree ID"=w170, "Name"=w169, "Tree Manager"=w174) -> ("Error Out"=w175:errorcluster, "Tree Manager"=w171:refnum<data-value>)  [unwired: 7 in]
                n60 = property on="Code Modules" class="Tree (strict)"("Active Item Tag"=w173, "ActiveColNum"=0 ("Active Cell:Active Column Number"), "Cell String"=w169) -> ()  [unwired: 2 in, 2 out]
              }
              frame True {
              }
            }
            n61 = call-poly <vilib>:"To Tree Data.vi"("String"=w158) -> ("String Tree Data"=w157:refnum<class "String.lvclass">)  [unwired: 10 in]
            n62 = call-poly <vilib>:"Set Polymorphic.vi"("Tree ID"=w160, "Error In"=w167, "Attribute Value"=w157, "Attribute Name"="Modified Desc", "Tree Manager"=w161) -> ()  [unwired: 4 in, 3 out]
            n63 = in-place {
              in-place-border: w160 -> [w179]
              n64 = in-place-cluster #1(w163) -> ("Unsaved Items"=w180:variant)
              n65 = Set Variant Attribute(Variant=w180, name=w179, value=TRUE) -> (Variant out=w178:variant)  [unwired: 1 in, 2 out]
              n66 = in-place-cluster #1("Unsaved Items"=w178) -> (w162:T2)
            }
          }
          event "Load XML File": Value Change {
            n67 = event-data() -> ()  [unwired: 1 in, 1 out]
            n68 = call <vilib>:"Set Busy.vi"("error in (no error)"=w219) -> ("error out"=w187:errorcluster)  [unwired: 9 in, 1 out]
            n69 = Unbundle By Name(w205) -> ("XML Tree"=w208:refnum<data-value>)
            n70 = call <vilib>:"Release Tree Manager.vi"("Error In"=w187, "Tree"=w208) -> ("Error Out"=w218:errorcluster)  [unwired: 9 in]
            n71 = control-ref of="XML File"() -> (w189:refnum<vi>)
            n72 = call <vilib>:"Clear Errors.vi"("error in (no error)"=w218) -> ("error out"=w217:errorcluster)  [unwired: 5 in, 1 out]
            n73 = call <vilib>:"Obtain Tree Manager.vi"("Error In"=w217) -> ("Error Out"=w215:errorcluster, "Tree"=w207:refnum<data-value>)  [unwired: 9 in]
            n74 = property class="Tree (strict)"(reference=w189) -> (reference out=w197:refnum<vi>, error out=w211:errorcluster, "OwningVI"=w195:refnum<vi>)  [unwired: 1 in]
            n75 = call-poly <vilib>:"Load.vi"("path to XML document"="XML File Path", "error in (no error)"=w215) -> ("DOM document out"=w203:refnum<k20>, "error out"=w216:errorcluster)  [unwired: 11 in, 1 out]
            n76 = call "Recursive XML Parse - Specific.vi"("error in (no error)"=w216, "DOM document in"=w203, "Tree"=w207) -> ("Tree Manager"=w193:refnum<data-value>)  [unwired: 7 in, 1 out]
            n77 = property class="VI"(reference=w195, error in=w211) -> (error out=w212:errorcluster, "Panel"=w196:refnum<vi>)  [unwired: 1 out]
            n78 = property class="Pnl"(reference=w196, error in=w212, "DeferPanUpdts"=TRUE ("Defer Panel Updates")) -> (reference out=w201:refnum<vi>, error out=w213:errorcluster)
            n79 = invoke class="Tree (strict)" method="Edit Tree Items.Delete"(reference=w197, error in=w213) -> (reference out=w200:refnum<vi>, error out=w209:errorcluster)  [unwired: 3 in, 3 out]
            n80 = call-poly <vilib>:"List Polymorphic.vi"("Error In"=w209, "Tree"=w193) -> ("Error Out"=w210:errorcluster, "Tree"=w192:refnum<data-value>, "Roots IDs"=w191:string[])  [unwired: 6 in, 1 out]
            n81 = Index Array(array=w191) -> (element=w190:string)  [unwired: 1 in]
            n82 = call <vilib>:"Show Tree.vi"("Root ID"=w190, "Error In"=w210, "Tree"=w192) -> ("Error Out"=w214:errorcluster, "Items Out"=w202:T5, "Tree"=w194:refnum<data-value>)  [unwired: 6 in]
            n83 = invoke class="Tree (strict)" method="Edit Tree Items.Add Multiple Items to End"(reference=w200, error in=w214, "Items"=w202) -> (reference out=w182:refnum<vi>, error out=w184:errorcluster)  [unwired: 1 in, 2 out]
            n84 = Bundle By Name(cluster=w205, "XML Tree"=w194) -> (w206:T2)
            n85 = invoke class="Tree (strict)" method="Edit Tree Items.Sort Children"(reference=w182, error in=w184, "Sort Recursively"=TRUE ("Sort Recursively?")) -> (error out=w183:errorcluster)  [unwired: 5 in, 7 out]
            n86 = property class="Pnl"(reference=w201, error in=w183, "DeferPanUpdts"=FALSE ("Defer Panel Updates")) -> (error out=w185:errorcluster)  [unwired: 1 out]
            n87 = call <vilib>:"Unset Busy.vi"("error in (no error)"=w185) -> ("error out"=w186:errorcluster)  [unwired: 10 in]
          }
          event "Copy": Value Change {
            n88 = event-data() -> ()  [unwired: 1 in, 6 out]
            n89 = property on="Selected XML Data" class="Str"() -> ("Value"=w221:string)  [unwired: 2 in, 2 out]
            n90 = property on="Element Description" class="Str"("Val(Sgnl)"=w221) -> ()  [unwired: 2 in, 2 out]
          }
          event "Code Modules": Value Change {
            # "Get modified description if existing"
            n91 = event-data() -> ("NewVal"=w234:string)  [unwired: 1 in, 4 out]
            n92 = Unbundle By Name(w235) -> ("LabVIEW Tree"=w227:refnum<data-value>)
            n93 = call <vilib>:"Tag to Tree ID and Attribute Name.vi"("Tag"=w234) -> ("Tree ID"=w231:string)  [unwired: 8 in, 2 out]
            n94 = call-poly <vilib>:"Get Polymorphic.vi"("Tree ID"=w231, "Attribute Name"="Modified Desc", "Tree Manager"=w227) -> ("Error Out"=w225:errorcluster, "Attribute Value"=w233:refnum<class "Tree Data.lvclass">, "Found?"=w230:bool)  [unwired: 5 in, 1 out]
            n95 = call-poly <vilib>:"Get Polymorphic.vi"("Tree ID"=w231, "Tree Manager"=w227) -> ("Meta Data"=w228:string)  [unwired: 7 in, 2 out]
            n96 = call <vilib>:"Clear Errors.vi"("error in (no error)"=w225) -> ()  [unwired: 5 in, 2 out]
            n97 = call-poly <vilib>:"From Tree Data.vi"("Tree Data"=w233) -> ("String"=w229:string)  [unwired: 10 in]
            n98 = Select(t=w229, s=w230, f=w228) -> (s? t:f=w226:string)
            n99 = property on="Element Description" class="Str"("Value"=w226) -> ()  [unwired: 2 in, 2 out]
          }
          event "XML File": Value Change {
            n100 = event-data() -> ("NewVal"=w238:string)  [unwired: 1 in, 4 out]
            n101 = Unbundle By Name(w242) -> ("XML Tree"=w241:refnum<data-value>)
            n102 = call <vilib>:"Tag to Tree ID and Attribute Name.vi"("Tag"=w238) -> ("Tree ID"=w240:string)  [unwired: 8 in, 2 out]
            n103 = call-poly <vilib>:"Get Polymorphic.vi"("Tree ID"=w240, "Tree Manager"=w241) -> ("Meta Data"=→"Selected XML Data":string)  [unwired: 7 in, 2 out]
          }
          event "Cancel All": Value Change {
            w250 = T1[] [enum."Update Code Modules Display"] items=["<Init>", "Wait for Event", "Update Code Modules Display", "Save Files", "<Shutdown>"]
            n104 = event-data() -> ()  [unwired: 1 in, 6 out]
            n105 = Unbundle By Name(w252) -> ("Unsaved Items"=w247:variant, "LabVIEW Tree"=w251:refnum<data-value>)
            n106 = Get Variant Attribute(Variant=w247) -> (names=w246:string[])  [unwired: 3 in, 3 out]
            n107 = for {
              tunnel: w246 -> [w257] mode=indexing
              tunnel: w251 -> [w262]
              tunnel: [w254] -> w248
              n108 = call-poly <vilib>:"Get Polymorphic.vi"("Tree ID"=w257, "Tree Manager"=w262) -> ("Error Out"=w263:errorcluster, "Name"=w260:string, "Tree Manager"=w261:refnum<data-value>)  [unwired: 7 in]
              n109 = String Subset(string=w260, offset (0)=1) -> (substring=w259:string)  [unwired: 1 in]
              n110 = call-poly <vilib>:"Set Polymorphic.vi"("Tree ID"=w257, "Error In"=w263, "Name"=w259, "Tree Manager"=w261) -> ("Error Out"=w264:errorcluster, "Tree Manager"=w256:refnum<data-value>)  [unwired: 6 in]
              n111 = call-poly <vilib>:"Delete Polymorphic.vi"("Tree ID"=w257, "Error In"=w264, "Attribute Name"="Modified Desc", "Tree Manager"=w256) -> ("Error Out"=w254:errorcluster)  [unwired: 4 in, 3 out]
            }
            n112 = property on="Code Modules" class="Tree (strict)"(error in=w248) -> ("Value"=w249:string)  [unwired: 1 in, 2 out]
            n113 = property on="Code Modules" class="Tree (strict)"("Val(Sgnl)"=w249) -> ()  [unwired: 2 in, 2 out]
            n114 = Bundle By Name(cluster=w252, "Unsaved Items"=variant) -> (w245:T2)
          }
          event "Cancel": Value Change {
            w278 = T1[] [enum."Update Code Modules Display"] items=["<Init>", "Wait for Event", "Update Code Modules Display", "Save Files", "<Shutdown>"]
            n115 = event-data() -> ()  [unwired: 1 in, 6 out]
            n116 = property on="Code Modules" class="Tree (strict)"() -> ("Value"=w266:string)  [unwired: 2 in, 2 out]
            n117 = Unbundle By Name(w267) -> ("LabVIEW Tree"=w279:refnum<data-value>)
            n118 = in-place {
              in-place-border: w266 -> [w281]
              n119 = in-place-cluster #2(w267) -> ("Unsaved Items"=w283:variant)
              n120 = Delete Variant Attribute(6:w281, 7:w283) -> (3:w282:variant)  [unwired: 1 in, 2 out]
              n121 = in-place-cluster #2("Unsaved Items"=w282) -> (w265:T2)
            }
            n122 = call-poly <vilib>:"Get Polymorphic.vi"("Tree ID"=w266, "Tree Manager"=w279) -> ("Error Out"=w274:errorcluster, "Name"=w272:string, "Tree Manager"=w273:refnum<data-value>)  [unwired: 7 in]
            n123 = String Subset(string=w272, offset (0)=1) -> (substring=w271:string)  [unwired: 1 in]
            n124 = call-poly <vilib>:"Set Polymorphic.vi"("Tree ID"=w266, "Error In"=w274, "Name"=w271, "Tree Manager"=w273) -> ("Error Out"=w275:errorcluster, "Tree Manager"=w269:refnum<data-value>)  [unwired: 6 in]
            n125 = call-poly <vilib>:"Delete Polymorphic.vi"("Tree ID"=w266, "Error In"=w275, "Attribute Name"="Modified Desc", "Tree Manager"=w269) -> ("Error Out"=w276:errorcluster)  [unwired: 4 in, 3 out]
            n126 = property on="Code Modules" class="Tree (strict)"(error in=w276) -> ("Value"=w277:string)  [unwired: 1 in, 2 out]
            n127 = property on="Code Modules" class="Tree (strict)"("Val(Sgnl)"=w277) -> ()  [unwired: 2 in, 2 out]
          }
          event "Apply": Value Change {
            w288 = T1[] [enum."Save Files", enum."Update Code Modules Display"] items=["<Init>", "Wait for Event", "Update Code Modules Display", "Save Files", "<Shutdown>"]
            n128 = event-data() -> ()  [unwired: 1 in, 6 out]
            n129 = property on="Code Modules" class="Tree (strict)"() -> ("Value"=w285:string)  [unwired: 2 in, 2 out]
            n130 = Build Array(w285) -> (w284:string[])
            n131 = Bundle By Name(cluster=w287, "Items to Save"=w284) -> (w286:T2)
          }
          event "Apply All Unsaved": Value Change {
            w294 = T1[] [enum."Save Files", enum."Update Code Modules Display"] items=["<Init>", "Wait for Event", "Update Code Modules Display", "Save Files", "<Shutdown>"]
            n132 = event-data() -> ()  [unwired: 1 in, 6 out]
            n133 = Unbundle By Name(w292) -> ("Unsaved Items"=w291:variant)
            n134 = Get Variant Attribute(Variant=w291) -> (names=w290:string[])  [unwired: 3 in, 3 out]
            n135 = Bundle By Name(cluster=w292, "Items to Save"=w290) -> (w293:T2)
          }
        }
      }
      frame "Update Code Modules Display" {
        n136 = control-ref of="Code Modules"() -> (w301:refnum<vi>)
        n137 = Unbundle By Name(w315) -> ("Control Strings"=w298:string[], "LabVIEW Tree"=w304:refnum<data-value>)
        n138 = property class="Tree (strict)"(reference=w301) -> (reference out=w309:refnum<vi>, error out=w319:errorcluster, "OwningVI"=w307:refnum<vi>)  [unwired: 1 in]
        n139 = property class="VI"(reference=w307, error in=w319) -> (error out=w320:errorcluster, "Panel"=w308:refnum<vi>)  [unwired: 1 out]
        n140 = property class="Pnl"(reference=w308, error in=w320, "DeferPanUpdts"=TRUE ("Defer Panel Updates")) -> (reference out=w313:refnum<vi>, error out=w321:errorcluster)
        n141 = invoke class="Tree (strict)" method="Edit Tree Items.Delete"(reference=w309, error in=w321) -> (reference out=w312:refnum<vi>, error out=w317:errorcluster)  [unwired: 3 in, 3 out]
        n142 = call-poly <vilib>:"List Polymorphic.vi"("Error In"=w317, "Tree"=w304) -> ("Error Out"=w318:errorcluster, "Tree"=w305:refnum<data-value>, "Roots IDs"=w306:string[])  [unwired: 6 in, 1 out]
        n143 = Index Array(array=w306) -> (element=w303:string)  [unwired: 1 in]
        n144 = call <vilib>:"Show Tree.vi"("Root ID"=w303, "Error In"=w318, "Tree"=w305) -> ("Error Out"=w322:errorcluster, "Items Out"=w314:T5)  [unwired: 6 in, 1 out]
        n145 = invoke class="Tree (strict)" method="Edit Tree Items.Add Multiple Items to End"(reference=w312, error in=w322, "Items"=w314) -> (reference out=w302:refnum<vi>, error out=w316:errorcluster)  [unwired: 1 in, 2 out]
        n146 = invoke on="Invoke Node" class="Tree (strict)" method="Edit Tree Items.Sort Children"(reference=w302, error in=w316) -> (reference out=w300:refnum<vi>, error out=w299:errorcluster)  [unwired: 6 in, 6 out]
        n147 = for {
          tunnel: w300 -> [w328]
          tunnel: w299 -> [w327]
          tunnel: w298 -> [w326] mode=indexing
          tunnel: [w324] -> w297
          n148 = invoke on="Invoke Node" class="Tree (strict)" method="Open/Close.Item"(reference=w328, error in=w327, "tag"=w326, "Open"=FALSE ("Open?")) -> (error out=w324:errorcluster)  [unwired: 1 in, 4 out]
        }
        n149 = property class="Pnl"(reference=w313, error in=w297, "DeferPanUpdts"=FALSE ("Defer Panel Updates")) -> ()  [unwired: 2 out]
      }
      frame "Save Files" {
        n150 = Unbundle By Name(w334) -> ("LabVIEW Tree"=w335:refnum<data-value>, "Items to Save"=w332:string[])
        n151 = for {
          tunnel: w335 -> [w347]
          shift-right: [w338] -> w333
          shift-left: w334 -> [w339]
          tunnel: w332 -> [w337] mode=indexing
          w340 = "Modified Desc" ("Attribute Name")
          n152 = call <vilib>:"Tag to Tree ID and Attribute Name.vi"("Tag"=w337) -> ("Tree ID"=w341:string)  [unwired: 8 in, 2 out]
          n153 = call-poly <vilib>:"Get Polymorphic.vi"("Tree ID"=w341, "Attribute Name"=w340, "Tree Manager"=w347) -> ("Error Out"=w346:errorcluster, "Attribute Value"=w343:refnum<class "Tree Data.lvclass">, "Found?"=w345:bool, "Tree Manager"=w344:refnum<data-value>)  [unwired: 5 in]
          n154 = call-poly <vilib>:"From Tree Data.vi"("Tree Data"=w343) -> ("String"=w342:string)  [unwired: 10 in]
          n155 = call <vilib>:"Clear Errors.vi"("error in (no error)"=w346) -> ()  [unwired: 5 in, 2 out]
          n156 = case shown="True" w345 {
            tunnel: w344 -> [_ w366]
            tunnel: w342 -> [_ w349]
            tunnel: w339 -> [w348 w369]
            tunnel: [w348 w368] -> w338
            tunnel: w341 -> [_ w367]
            tunnel: w341 -> [_ w359]
            tunnel: w340 -> [_ w352]
            frame False {
            }
            frame True {
              n157 = call-poly <vilib>:"Get Polymorphic.vi"("Tree ID"=w359, "Attribute Name"="VI Ref", "Tree Manager"=w366) -> ("Attribute Value"=w361:variant, "Found?"=w360:bool, "Tree Manager"=w356:refnum<data-value>)  [unwired: 5 in, 1 out]
              n158 = case shown="True" w360 {
                tunnel: w361 -> [_ w390]
                tunnel: w359 -> [w378 w389]
                tunnel: [w378 w389] -> w351
                tunnel: [w374 w385] -> w358
                tunnel: w356 -> [w377 w384]
                tunnel: [w376 w384] -> w355
                tunnel: w349 -> [w372 w386]
                frame False {
                  n159 = call-poly <vilib>:"Get Polymorphic.vi"("Tree ID"=w378, "Attribute Name"="Ctrl Ref", "Tree Manager"=w377) -> ("Attribute Value"=w373:variant, "Found?"=w371:bool, "Tree Manager"=w376:refnum<data-value>)  [unwired: 5 in, 1 out]
                  n160 = case shown="True" w371 {
                    tunnel: [_ w381] -> w374
                    tunnel: w373 -> [_ w380]
                    tunnel: w372 -> [_ w379]
                    frame False {
                    }
                    frame True {
                      n161 = Variant To Data(type=refnum<vi> refnum ("References"), Variant=w380) -> (data=w382:refnum<vi>)  [unwired: 1 in, 1 out]
                      n162 = property class="Ctl"(reference=w382, "Desc"=w379) -> ("OwningVI"=w381:refnum<vi>)  [unwired: 1 in, 2 out]
                    }
                  }
                }
                frame True {
                  n163 = Variant To Data(type=refnum<vi> refnum ("reference out"), Variant=w390) -> (data=w387:refnum<vi>)  [unwired: 1 in, 1 out]
                  n164 = property class="VI"(reference=w387, "Description"=w386) -> (reference out=w385:refnum<vi>)  [unwired: 1 in, 1 out]
                }
              }
              n165 = in-place {
                in-place-border: w367 -> [w391]
                n166 = in-place-cluster #3(w369) -> ("Unsaved Items"=w393:variant)
                n167 = Delete Variant Attribute(6:w391, 7:w393) -> (3:w392:variant)  [unwired: 1 in, 2 out]
                n168 = in-place-cluster #3("Unsaved Items"=w392) -> (w368:T2)
              }
              n169 = Not A Number/Path/Refnum?(number/path/refnum=w358) -> (NaN/Path/Refnum?=w357:bool)
              n170 = case shown="True" w357 {
                tunnel: w358 -> [w370 _]
                frame False {
                  n171 = invoke class="VI" method="Save.Instrument"(reference=w370) -> ()  [unwired: 5 in, 6 out]
                }
                frame True {
                }
              }
              n172 = call-poly <vilib>:"Get Polymorphic.vi"("Tree ID"=w351, "Tree Manager"=w355) -> ("Name"=w363:string, "Tree Manager"=w365:refnum<data-value>)  [unwired: 7 in, 1 out]
              n173 = String Subset(string=w363, offset (0)=1) -> (substring=w362:string)  [unwired: 1 in]
              n174 = call-poly <vilib>:"Set Polymorphic.vi"("Tree ID"=w351, "Name"=w362, "Tree Manager"=w365) -> ("Tree Manager"=w353:refnum<data-value>)  [unwired: 7 in, 1 out]
              n175 = call-poly <vilib>:"Delete Polymorphic.vi"("Tree ID"=w351, "Attribute Name"=w352, "Tree Manager"=w353) -> ("Tree Manager"=w350:refnum<data-value>)  [unwired: 5 in, 3 out]
              n176 = call-poly <vilib>:"Set Polymorphic.vi"("Tree ID"=w351, "Meta Data"=w349, "Tree Manager"=w350) -> ()  [unwired: 7 in, 2 out]
            }
          }
        }
        n177 = Bundle By Name(cluster=w333, "Items to Save"=string[] []) -> (w331:T2)
      }
      frame "<Shutdown>" {
        n178 = Unbundle By Name(w401) -> ("LabVIEW Tree"=w395:refnum<data-value>, "XML Tree"=w394:refnum<data-value>, "References"=w396:refnum<vi>[])
        n179 = call <vilib>:"Release Tree Manager.vi"("Tree"=w395) -> ("Error Out"=w400:errorcluster)  [unwired: 10 in]
        n180 = call <vilib>:"Release Tree Manager.vi"("Tree"=w394) -> ("Error Out"=w399:errorcluster)  [unwired: 10 in]
        n181 = Close Reference(reference=w396) -> (error out=w398:errorcluster)  [unwired: 1 in]
        n182 = Merge Errors(w400, w399, w398) -> (w397:errorcluster)
        n183 = call <vilib>:"Clear Errors.vi"("error in (no error)"=w397) -> ()  [unwired: 5 in, 2 out]
      }
    }
  }
